vi "logger.vi"(4 "Annotation content":string, 5 "Annotation":bool, 6 "Name":string, 7 "error in":errorcluster, 8 "Data":variant, 9 "Configuration":string, 10 "Path to log":path) -> (0 "error out":errorcluster)   [LabVIEW 2019]
doc: "This VI creates text files or binary files depending on the type of sensor. \n**Text file:** \n - State sensor \n - Ultrasonic \n - Collision \n - Radar \n \n**Binary files:** \n - IMU \n - GPS \n - RPM \n - LiDAR \n - Semantic LiDAR \n - Camera \n\nIt also saves a text file for the camera annotation if the user sets the annotation flag to True."
uses:
  <vilib>/Utility/Data Type/NI_Data Type.lvlib
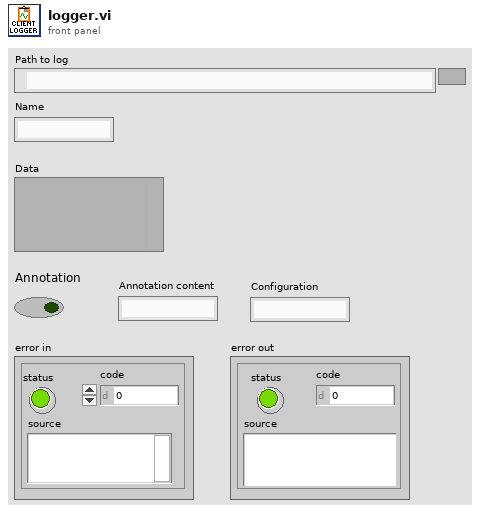
[diagram p1: front panel]
types:
  T1 = enum16{"big-endian, network order", "native, host order", "little-endian"}
  T2 = enum16{"open", "replace", "create", "open or create", "replace or create", "replace or create with confirmation"}
  T3 = typedef "NI_Data Type.lvlib/Data Type.ctl" = enum8{"Invalid Type", "Void", "I8", "I16", "I32", "I64", "U8", "U16", "U32", "U64", "Single Float", "Double Float", "Extended Float", "Single Complex", "Double Complex", "Extended Complex", "Enum U8", "Enum U16", "Enum U32", "Enum U64", "Single Float With Unit", "Double Float With Unit", "Extended Float With Unit", "Single Complex with Unit", "Double Complex with Unit", "Extended Complex with Unit", "Boolean", "String", "Path", "Picture", "Tag", "Array", "Cluster", "Variant", "LV Variant", "Waveform", "Timestamp", "Digital Waveform", "Digital Data", "ExpressData", "Refnum", "External Data", "VI", "Poly VI", "LabVIEW Class Instance", "Fixed Point", "Set Collection", "Map Collection"}
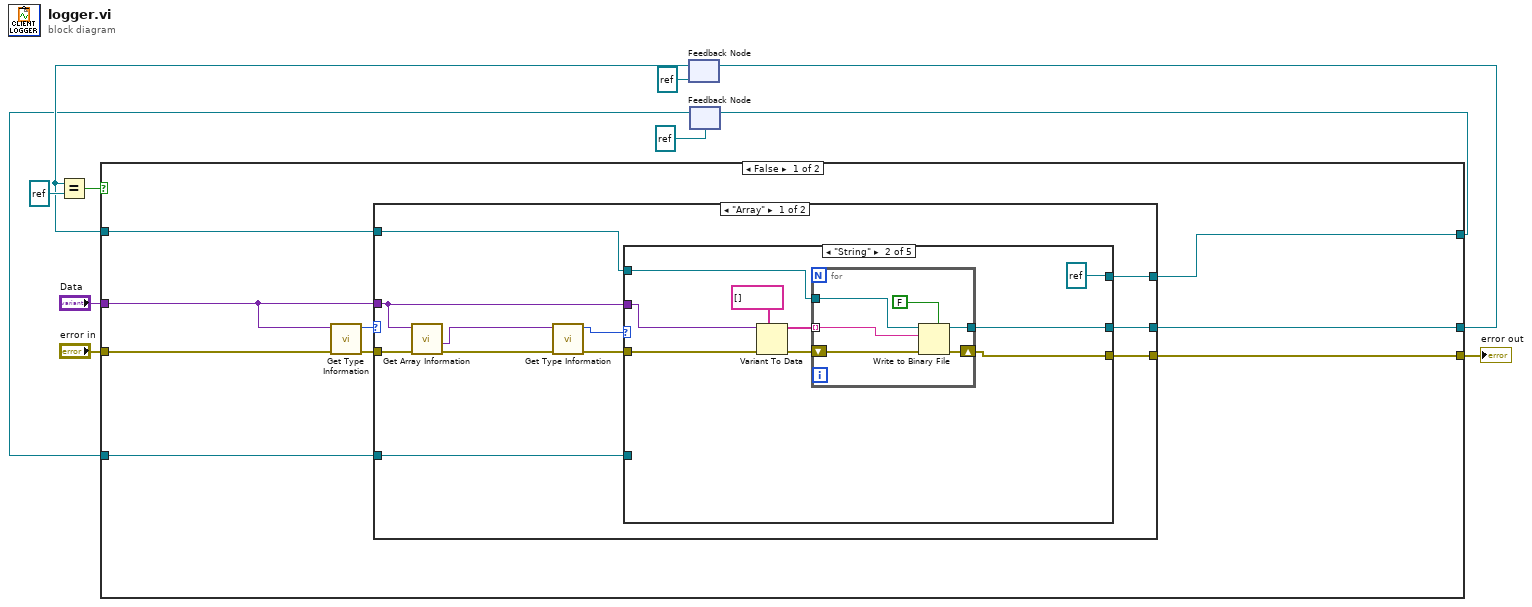
[diagram p0: block diagram]
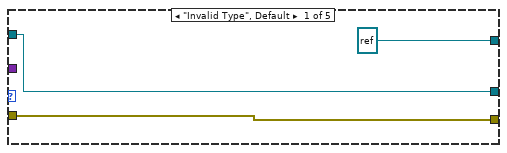
[diagram p2: hidden frame]
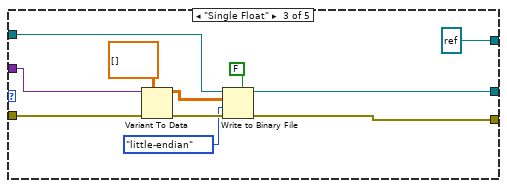
[diagram p3: hidden frame]
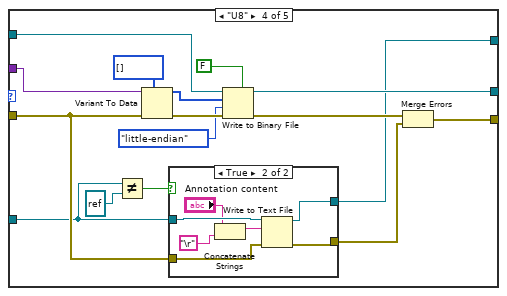
[diagram p4: hidden frame]
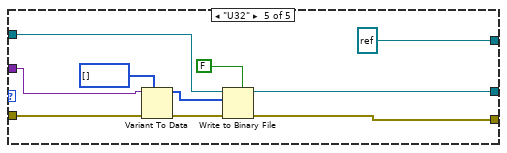
[diagram p6: hidden frame]
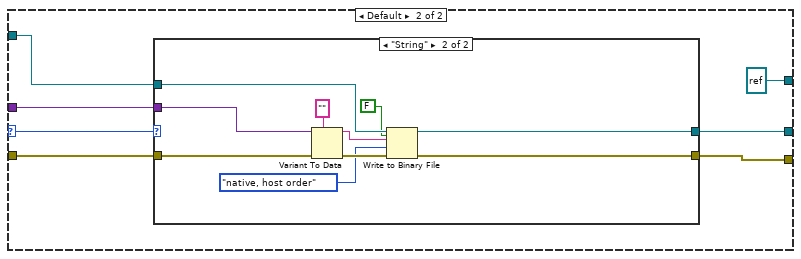
[diagram p7: hidden frame]
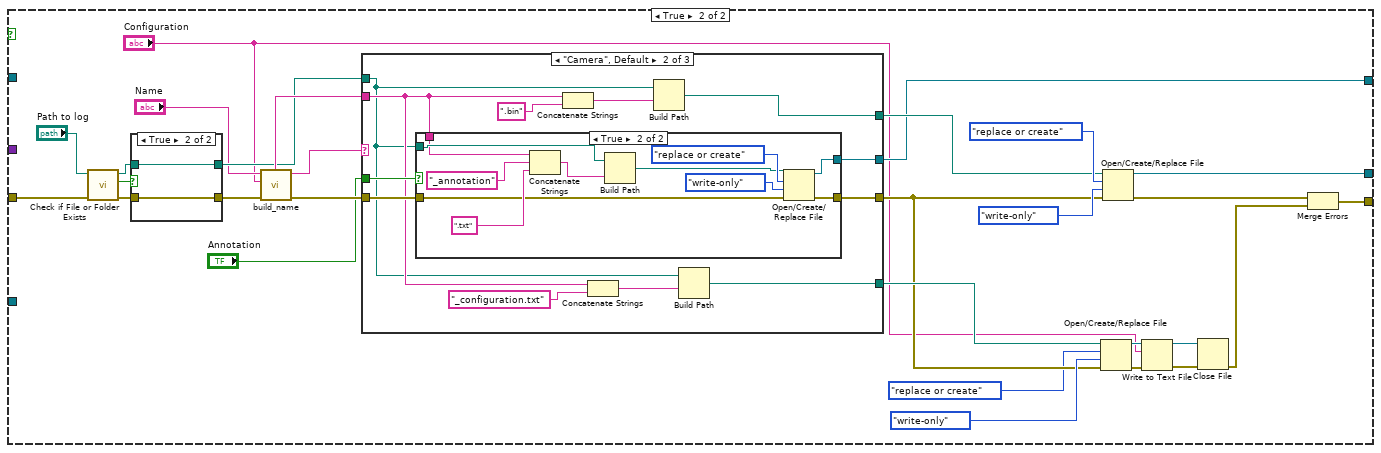
[diagram p9: hidden frame]
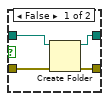
[diagram p10: hidden frame]
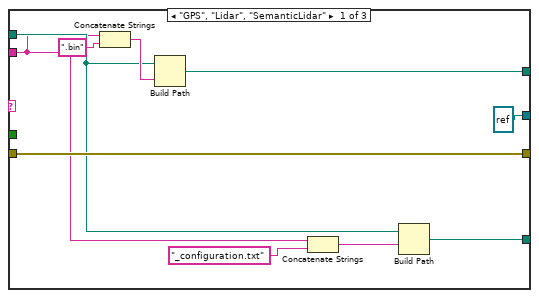
[diagram p11: hidden frame]
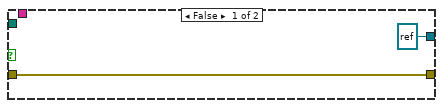
[diagram p12: hidden frame]
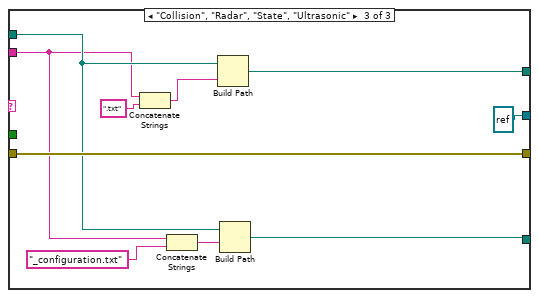
[diagram p13: hidden frame]
diagram:
  n1 = feedback #1(refnum<file> refnum ("refnum out")) -> (w6:refnum<file>)
  n2 = Equal?(x=w6, y=refnum<file> refnum ("refnum out")) -> (x = y?=w10:bool)
  n3 = feedback #2(refnum<file> refnum ("refnum out")) -> (w2:refnum<file>)
  n4 = case shown="False" w10 {
    tunnel: "error in" -> [w14 w135]
    tunnel: [w17 w128] -> w8
    tunnel: [w18 w141] -> w7
    tunnel: w6 -> [w15 _]
    tunnel: "Data" -> [w19 _]
    tunnel: [w12 w133] -> w3
    tunnel: w2 -> [w13 _]
    frame False {
      n5 = call <vilib>:"Get Type Information.vi"("error in (no error)"=w14, "variant"=w19) -> ("error out"=w16:errorcluster, "type"=w20:T3)  [unwired: 5 in, 3 out]
      n6 = case shown="\"Array\"" w20 {
        selector: w20 -> [_ w102]
        tunnel: w19 -> [w26 w101]
        tunnel: [w27 w100] -> w18
        tunnel: [w28 w99] -> w17
        tunnel: w16 -> [w24 w98]
        tunnel: w15 -> [w25 w97]
        tunnel: w13 -> [w22 _]
        tunnel: [w21 refnum<file> refnum ("refnum out")] -> w12
        frame "Array" {
          n7 = call <vilib>:"Get Array Information.vi"("error in (no error)"=w24, "variant"=w26) -> ("error out"=w23:errorcluster, "array element data type"=w30:variant)  [unwired: 6 in, 2 out]
          n8 = call <vilib>:"Get Type Information.vi"("error in (no error)"=w23, "variant"=w30) -> ("error out"=w29:errorcluster, "type"=w31:T3)  [unwired: 5 in, 3 out]
          n9 = case shown="\"String\"" w31 {
            tunnel: w26 -> [_ w43 w60 w76 w95]
            tunnel: [w33 w42 w59 w75 w94] -> w27
            tunnel: [w34 w41 w58 w67 w93] -> w28
            tunnel: w29 -> [w34 w39 w56 w68 w91]
            tunnel: w25 -> [w33 w36 w54 w71 w89]
            tunnel: w22 -> [_ _ _ w64 _]
            tunnel: [refnum<file> refnum ("refnum out") refnum<file> refnum ("refnum out") refnum<file> refnum ("refnum out") w65 refnum<file> refnum ("refnum out")] -> w21
            frame "Invalid Type", Default {
            }
            frame "String" {
              n10 = Variant To Data(error in=w39, type=string[] [], Variant=w43) -> (data=w38:string[], error out=w40:errorcluster)
              n11 = for {
                tunnel: [w49] -> w42
                tunnel: w38 -> [w46] mode=indexing
                tunnel: w36 -> [w45]
                shift-right: [w48] -> w41
                shift-left: w40 -> [w47]
                n12 = Write to Binary File(file (use dialog)=w45, data=w46, error in=w47, 5:FALSE ("prepend array or string size? (T)")) -> (refnum out=w49:refnum<file>, error out=w48:errorcluster)  [unwired: 2 in, 1 out]
              }
            }
            frame "Single Float" {
              n13 = Variant To Data(error in=w56, type=sgl[][] [] ("Data 2"), Variant=w60) -> (data=w55:sgl[][], error out=w57:errorcluster)
              n14 = Write to Binary File(file (use dialog)=w54, data=w55, error in=w57, 5:FALSE ("prepend array or string size? (T)"), 9:T1."little-endian" ("byte order (0:big-endian, network order)")) -> (refnum out=w59:refnum<file>, error out=w58:errorcluster)  [unwired: 1 in, 1 out]
            }
            frame "U8" {
              n15 = Not Equal?(x=w64, y=refnum<file> refnum) -> (x != y?=w62:bool)
              n16 = Variant To Data(error in=w68, type=u8[] [], Variant=w76) -> (data=w69:u8[], error out=w73:errorcluster)
              n17 = case shown="True" w62 {
                tunnel: w64 -> [w78 w85]
                tunnel: w68 -> [w77 w84]
                tunnel: [w77 w83] -> w66
                tunnel: [w78 w82] -> w65
                frame False {
                }
                frame True {
                  n18 = Concatenate Strings("Annotation content", "\r") -> (w81:string)
                  n19 = Write to Text File(file (use dialog)=w85, text=w81, error in=w84) -> (refnum out=w82:refnum<file>, error out=w83:errorcluster)  [unwired: 1 in, 1 out]
                }
              }
              n20 = Write to Binary File(file (use dialog)=w71, data=w69, error in=w73, 5:FALSE ("prepend array or string size? (T)"), 9:T1."little-endian" ("byte order (0:big-endian, network order)")) -> (refnum out=w75:refnum<file>, error out=w74:errorcluster)  [unwired: 1 in, 1 out]
              n21 = Merge Errors(w74, w66) -> (w67:errorcluster)
            }
            frame "U32" {
              n22 = Variant To Data(error in=w91, type=u32[] [], Variant=w95) -> (data=w87:u32[], error out=w92:errorcluster)
              n23 = Write to Binary File(file (use dialog)=w89, data=w87, error in=w92, 5:FALSE ("prepend array or string size? (T)")) -> (refnum out=w94:refnum<file>, error out=w93:errorcluster)  [unwired: 2 in, 1 out]
            }
          }
        }
        frame Default {
          n24 = case shown="\"String\"" w102 {
            tunnel: w101 -> [_ w114]
            tunnel: [w103 w113] -> w100
            tunnel: [w104 w112] -> w99
            tunnel: w98 -> [w104 w110]
            tunnel: w97 -> [w103 w108]
            frame "Invalid Type", Default {
            }
            frame "String" {
              n25 = Variant To Data(error in=w110, type="", Variant=w114) -> (data=w106:string, error out=w111:errorcluster)
              n26 = Write to Binary File(file (use dialog)=w108, data=w106, error in=w111, 5:FALSE ("prepend array or string size? (T)"), 9:T1."native, host order" ("byte order (0:big-endian, network order)")) -> (refnum out=w113:refnum<file>, error out=w112:errorcluster)  [unwired: 1 in, 1 out]
            }
          }
        }
      }
    }
    frame True {
      n27 = call <vilib>:"Check if File or Folder Exists.vi"("error in (no error)"=w135, "path"="Path to log") -> ("error out"=w137:errorcluster, "file or folder exists?"=w138:bool, "dup path"=w136:path)  [unwired: 7 in]
      n28 = case shown="True" w138 {
        tunnel: w137 -> [w147 w149]
        tunnel: [w146 w149] -> w118
        tunnel: w136 -> [w145 w148]
        tunnel: [w144 w148] -> w131
        frame False {
          n29 = Create Folder(path (use dialog)=w145, error in=w147) -> (created path=w144:path, error out=w146:errorcluster)  [unwired: 1 in, 1 out]
        }
        frame True {
        }
      }
      n30 = call "build_name.vi"("error in"=w118, "Configuration"="Configuration", "Name"="Name") -> ("error out"=w117:errorcluster, "Name"=w134:string, "Type"=w121:string)  [unwired: 2 in]
      n31 = case shown="\"Camera\", Default" w121 {
        tunnel: [w157 w169 w192] -> w139
        tunnel: w131 -> [w152 w160 w187]
        tunnel: w134 -> [w151 w161 w186]
        tunnel: [w156 w168 w191] -> w129
        tunnel: w117 -> [w156 w167 w191]
        tunnel: "Annotation" -> [_ w166 _]
        tunnel: [refnum<file> refnum ("refnum out") w165 refnum<file> refnum ("refnum out")] -> w133
        tunnel: [w150 w162 w185] -> w130
        frame "GPS", "Lidar", "SemanticLidar" {
          n32 = Concatenate Strings(w151, ".bin" ("string")) -> (w158:string)
          n33 = Build Path(base path=w152, name or relative path=w158) -> (appended path=w157:path)
          n34 = Concatenate Strings(w151, "_configuration.txt" ("string")) -> (w154:string)
          n35 = Build Path(base path=w152, name or relative path=w154) -> (appended path=w150:path)
        }
        frame "Camera", Default {
          n36 = case shown="True" w166 {
            tunnel: w160 -> [_ w182]
            tunnel: w161 -> [_ w181]
            tunnel: [w173 w177] -> w168
            tunnel: w167 -> [w173 w176]
            tunnel: [refnum<file> refnum ("refnum out") w174] -> w165
            frame False {
            }
            frame True {
              n37 = Concatenate Strings(w181, "_annotation" ("string"), ".txt" ("string")) -> (w184:string)
              n38 = Build Path(base path=w182, name or relative path=w184) -> (appended path=w175:path)
              n39 = Open/Create/Replace File(file path (use dialog)=w175, error in=w176, operation (0:open)=T2."replace or create", access (0:read/write)=enum16{"read/write", "read-only", "write-only"}."write-only") -> (refnum out=w174:refnum<file>, error out=w177:errorcluster)  [unwired: 2 in, 1 out]
            }
          }
          n40 = Concatenate Strings(w161, ".bin" ("string")) -> (w170:string)
          n41 = Concatenate Strings(w161, "_configuration.txt" ("string")) -> (w164:string)
          n42 = Build Path(base path=w160, name or relative path=w170) -> (appended path=w169:path)
          n43 = Build Path(base path=w160, name or relative path=w164) -> (appended path=w162:path)
        }
        frame "Collision", "Radar", "State", "Ultrasonic" {
          n44 = Concatenate Strings(w186, ".txt" ("string")) -> (w193:string)
          n45 = Concatenate Strings(w186, "_configuration.txt" ("string")) -> (w189:string)
          n46 = Build Path(base path=w187, name or relative path=w193) -> (appended path=w192:path)
          n47 = Build Path(base path=w187, name or relative path=w189) -> (appended path=w185:path)
        }
      }
      n48 = Open/Create/Replace File(file path (use dialog)=w130, error in=w129, operation (0:open)=T2."replace or create", access (0:read/write)=enum16{"read/write", "read-only", "write-only"}."write-only") -> (refnum out=w126:refnum<file>, error out=w127:errorcluster)  [unwired: 2 in, 1 out]
      n49 = Open/Create/Replace File(file path (use dialog)=w139, error in=w129, operation (0:open)=T2."replace or create", access (0:read/write)=enum16{"read/write", "read-only", "write-only"}."write-only") -> (refnum out=w141:refnum<file>, error out=w142:errorcluster)  [unwired: 2 in, 1 out]
      n50 = Write to Text File(file (use dialog)=w126, text="Configuration", error in=w127) -> (refnum out=w124:refnum<file>, error out=w125:errorcluster)  [unwired: 1 in, 1 out]
      n51 = Close File(refnum=w124, error in=w125) -> (error out=w123:errorcluster)  [unwired: 1 out]
      n52 = Merge Errors(w142, w123) -> (w128:errorcluster)
    }
  }
  "error out" <- w8
  n53 = feedback-in #1(w7) -> ()
  n54 = feedback-in #2(w3) -> ()
